vi "Set Transfer Valve.vi"(8 "error in (no error)":errorcluster, 9 "Interlock Chain.lvclass":refnum<class "Interlock Chain.lvclass">, 10 "Open? (False)":bool, 11 "Preparation Line in":refnum<class "Preparation Line.lvclass">) -> (0 "error out":errorcluster, 3 "Preparation Line out":refnum<class "Preparation Line.lvclass">)   [LabVIEW 2015, in "cRIO-Carbondioxide.lvlib" / "CO2-Actor.lvlib" / "Preparation Line.lvclass"]
uses:
  Preparation Line.lvclass
  Interlocks/Interlock Chain/Interlock Chain.lvclass
  <vilib>/ActorFramework/Actor/Actor.lvclass/Actor.ctl
  <vilib>/ActorFramework/Message Enqueuer/Message Enqueuer.lvclass/Message Enqueuer.ctl
  Preparation Line.lvclass/Preparation Line.ctl
  Valve Messages/Write Bit Field Msg/Write Bit Field Msg.lvclass/Write Bit Field Msg.ctl
  <vilib>/ActorFramework/Actor/Read Self Enqueuer.vi
  <vilib>/ActorFramework/Message Enqueuer/Enqueue.vi
  <vilib>/ActorFramework/Message Enqueuer/Init from Existing Queue.vi
  <vilib>/ActorFramework/Message Priority Queue/Priority Enqueue.vi
  <vilib>/ActorFramework/Actor/Actor.lvclass
  <vilib>/ActorFramework/Message Enqueuer/Message Enqueuer.lvclass
  Valve Messages/Write Bit Field Msg/Write Bit Field Msg.lvclass
  CO2 Actor/CO2 Actor.lvclass
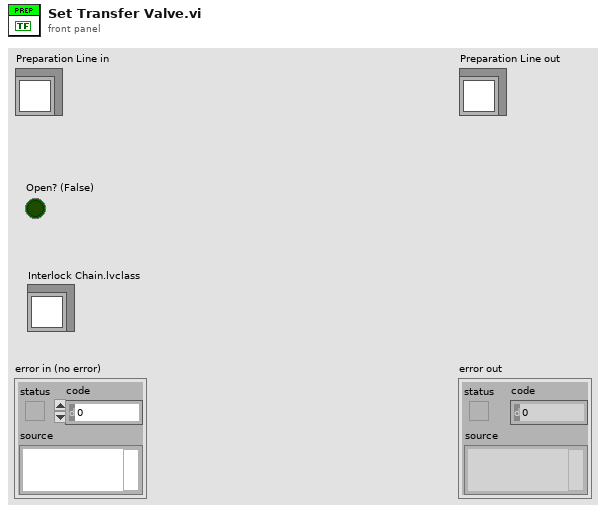
[diagram p1: front panel]
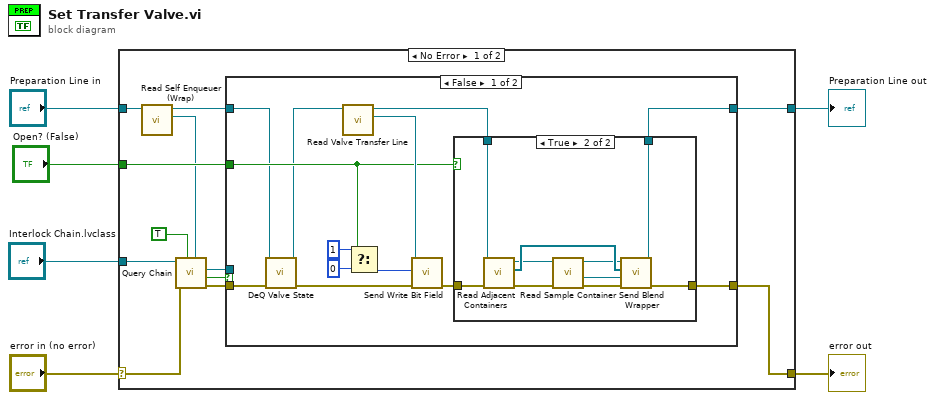
[diagram p0: block diagram]
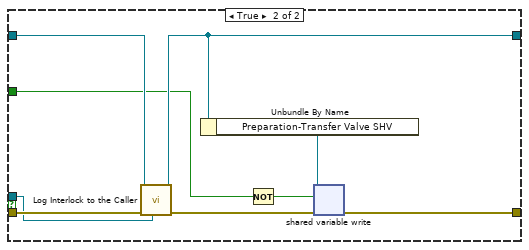
[diagram p3: hidden frame]
diagram:
  n1 = case shown="No Error" "error in (no error)" {
    selector: "error in (no error)" -> [w11 w54]
    tunnel: [w10 w54] -> w4
    tunnel: [w14 w53] -> w3
    tunnel: "Preparation Line in" -> [w9 w53]
    tunnel: "Interlock Chain.lvclass" -> [w18 _]
    tunnel: "Open? (False)" -> [w12 _]
    frame No Error {
      n2 = call "Read Self Enqueuer (Wrap).vi"("CO2 Actor in"=w9) -> ("Actor Framework:Message Enqueuer"=w7:refnum<class "Message Enqueuer.lvclass">, "CO2 Actor out"=w8:refnum<class "Preparation Line.lvclass">)  [unwired: 9 in]
      n3 = call "Query Chain.vi"("Caller Enqueuer"=w7, "Close Connections (F)"=TRUE, "error in (no error)"=w11, "Interlock Chain"=w18) -> ("error out"=w16:errorcluster, "Interlock?"=w13:bool, "Interlock out"=w15:refnum<class "Interlock.lvclass">)  [unwired: 2 in, 3 out]
      n4 = case shown="False" w13 {
        tunnel: w16 -> [w22 w52]
        tunnel: w15 -> [_ w51]
        tunnel: w8 -> [w20 w50]
        tunnel: [w25 w49] -> w14
        tunnel: w12 -> [w23 w46]
        tunnel: [w24 w44] -> w10
        frame False {
          n5 = call "DeQ Valve State.vi"("error in (no error)"=w22, "Preparation Line in"=w20) -> ("error out"=w21:errorcluster, "Preparation Line out"=w19:refnum<class "Preparation Line.lvclass">)  [unwired: 6 in, 2 out]
          n6 = call "Read Valve Transfer Line.vi"("Preparation Line in"=w19) -> ("Actor Framework:Message Enqueuer"=w27:refnum<class "Message Enqueuer.lvclass">, "Preparation Line out"=w26:refnum<class "Preparation Line.lvclass">)  [unwired: 9 in]
          n7 = Select(t=u16 1, s=w23, f=u16 0 ("Bit Field")) -> (s? t:f=w29:u16)
          n8 = call "Send Write Bit Field.vi"("error in (no error)"=w21, "Bit Field"=w29, "Message Enqueuer"=w27) -> ("error out"=w28:errorcluster)  [unwired: 5 in, 3 out]
          n9 = case shown="True" w23 {
            tunnel: w28 -> [w32 w43]
            tunnel: w26 -> [w33 w36]
            tunnel: [w33 w35] -> w25
            tunnel: [w32 w34] -> w24
            frame False {
            }
            frame True {
              n10 = call "Read Adjacent Containers.vi"("error in (no error)"=w43, "Preparation Line in"=w36) -> ("error out"=w42:errorcluster, "Adjacent Containers"=w39:refnum<class "Message Enqueuer.lvclass">[], "Preparation Line out"=w38:refnum<class "Preparation Line.lvclass">)  [unwired: 7 in]
              n11 = call "Read Sample Container.vi"("error in (no error)"=w42, "Preparation Line in"=w38) -> ("error out"=w41:errorcluster, "Sample"=w40:refnum<class "Sample.lvclass">, "Preparation Line out"=w37:refnum<class "Preparation Line.lvclass">)  [unwired: 6 in, 1 out]
              n12 = call-dynamic "Send Blend Wrapper.vi"("error in (no error)"=w41, "Sample to Blend"=w40, "Send to"=w39, "CO2 Actor in"=w37) -> ("error out"=w34:errorcluster, "CO2 Actor out"=w35:refnum<class "Preparation Line.lvclass">)  [unwired: 6 in]
            }
          }
        }
        frame True {
          n13 = call-dynamic "Log Interlock to the Caller.vi"("Interlock in"=w51, "error in (no error)"=w52, "CO2 Actor in"=w50) -> ("error out"=w48:errorcluster, "CO2 Actor out"=w49:refnum<class "Preparation Line.lvclass">)  [unwired: 7 in]
          n14 = Unbundle By Name(w49) -> ("Preparation-Transfer Valve SHV"=w47:refnum<k21>)
          n15 = Not(x=w46) -> (.not. x?=w45:bool)
          n16 = shared-variable-write(w47, w48, w45) -> (w44:errorcluster)  [unwired: 1 out]
        }
      }
    }
    frame Error {
    }
  }
  "error out" <- w4
  "Preparation Line out" <- w3
